vi "OxITC503 _Utility_ Calculate ITC Temp.vi"(1 "Sensor 3":dbl format="%.2f", 2 "Sensor 2":dbl format="%.2f") -> (0 "Temperature (K)":dbl format="%.2f")   [LabVIEW 2013]
panel:
  out "ss3":dbl format="%.2f"
  out "ss2":dbl format="%.2f"
  out "dt":dbl format="%.2f"
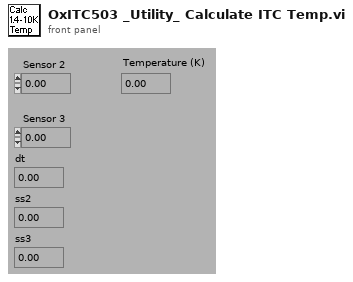
[diagram p1: front panel]
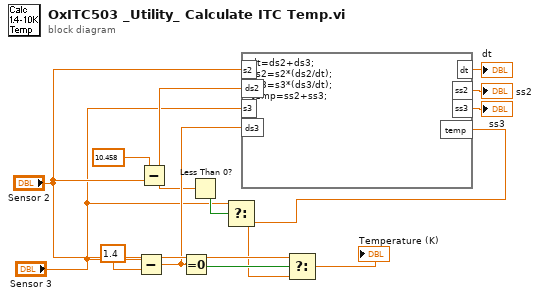
[diagram p0: block diagram]
diagram:
  n1 = Subtract(x="Sensor 3", y=1.4) -> (x-y=w10:dbl)
  n2 = Subtract(x=10.458 ("y"), y="Sensor 2") -> (x-y=w8:dbl)
  n3 = Equal To 0?(x=w10) -> (x = 0?=w13:bool)
  n4 = Less Than 0?(x=w8) -> (x < 0?=w7:bool)
  n5 = formula code="dt=ds2+ds3;\nss2=s2*(ds2/dt);\nss3=s3*(ds3/dt);\ntemp=ss2+ss3;"("s2"="Sensor 2", "s3"="Sensor 3", "ds2"=w8, "ds3"=w10) -> ("dt"=→"dt":dbl, "ss2"=→"ss2":dbl, "ss3"=→"ss3":dbl, "temp"=w5:dbl)
  n6 = Select(t="Sensor 3", s=w7, f=w5) -> (s? t:f=w4:dbl)
  n7 = Select(t="Sensor 2", s=w13, f=w4) -> (s? t:f=→"Temperature (K)":dbl)
